vi "PIN READ.vi"(8 "error in (no error)":errorcluster, 11 "NXP in":refnum<class "NXP.lvclass">) -> (0 "error out":errorcluster, 2 "VALUE":string, 3 "NXP out":refnum<class "NXP.lvclass">)   [LabVIEW 2020, in "NXP.lvclass"]
uses:
  NXP.lvclass
  NXP.lvclass/NXP.ctl
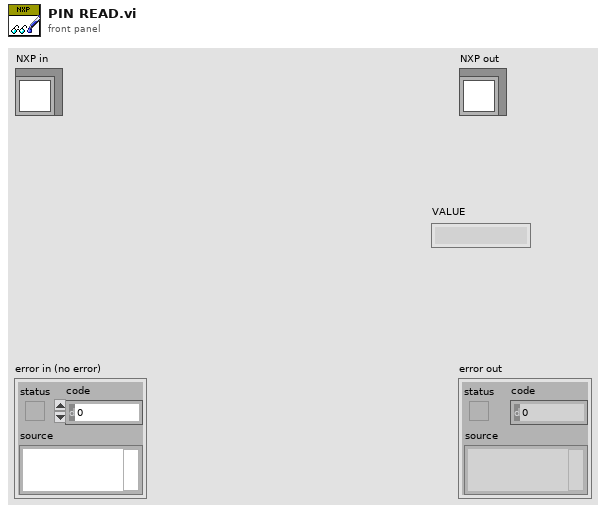
[diagram p1: front panel]
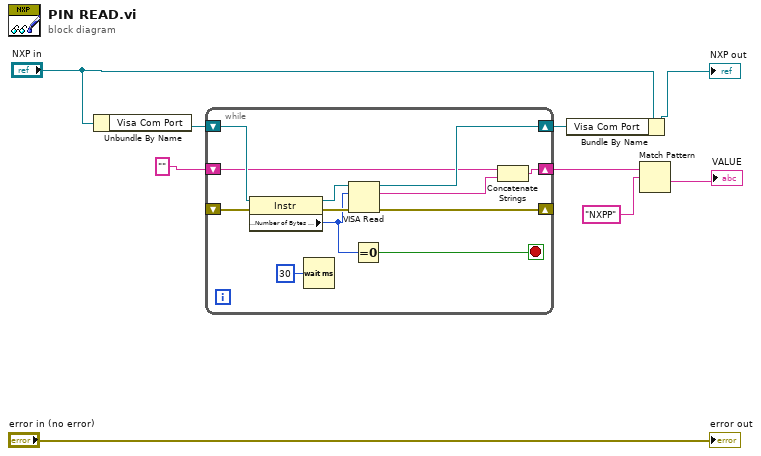
[diagram p0: block diagram]
diagram:
  n1 = Unbundle By Name("NXP in") -> ("Visa Com Port"=w7:refnum<visa-resource-name>)
  n2 = while {
    shift-right: [w21] -> _
    shift-left: _ -> [w16]
    shift-right: [w20] -> w8
    shift-left: w7 -> [w18]
    shift-right: [w12] -> w4
    shift-left: "" -> [w11]
    stop <- w13 stop-if-true
    n3 = property class="Instr"(reference=w18, error in=w16) -> (reference out=w17:refnum<visa-resource-name>, error out=w15:errorcluster, "Serial Settings:Number of Bytes at Serial Port"=w14:u32)
    n4 = Wait (ms)(milliseconds to wait=u32 30) -> ()  [unwired: 1 out]
    n5 = VISA Read(VISA resource name=w17, byte count=w14, error in (no error)=w15) -> (VISA resource name out=w20:refnum<visa-resource-name>, read buffer=w19:string, error out=w21:errorcluster)  [unwired: 1 out]
    n6 = Equal To 0?(x=w14) -> (x = 0?=w13:bool)
    n7 = Concatenate Strings(w11, w19) -> (w12:string)
  }
  n8 = Bundle By Name(cluster="NXP in", "Visa Com Port"=w8) -> (→"NXP out":refnum<class "NXP.lvclass">)
  n9 = Match Pattern(string=w4, regular expression="NXPP") -> (after substring=→"VALUE":string)  [unwired: 1 in, 3 out]
  "error out" <- "error in (no error)"
